vi "LVClasse_SurfaceFloatWithPupil Read SurfaceFloatWithPupil.vi"(8 "error in (no error)":errorcluster, 11 "SurfaceFloatWithPupil in":refnum<class "SurfaceFloatWithPupil.lvclass">) -> (0 "error out":errorcluster, 2 "SurfaceFloatWithPupil":T1, 3 "SurfaceFloatWithPupil out":refnum<class "SurfaceFloatWithPupil.lvclass">)   [LabVIEW 2020, in "SurfaceFloatWithPupil.lvclass"]
uses:
  SurfaceFloatWithPupil.lvclass
  ClassID.ctl
  SurfaceFloatWithPupil.lvclass/SurfaceFloatWithPupil.ctl
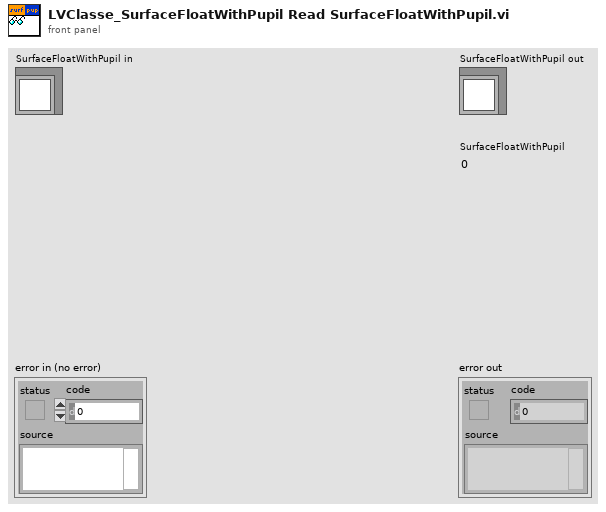
[diagram p1: front panel]
types:
  T1 = typedef "ClassID.ctl" = i64
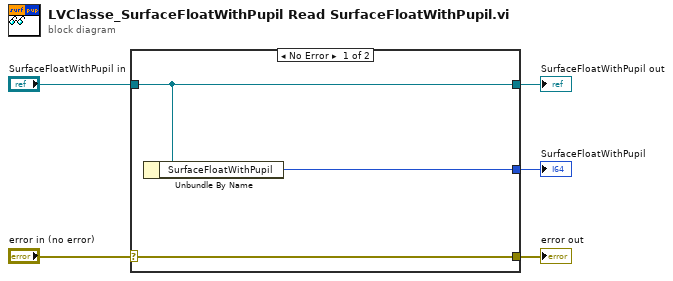
[diagram p0: block diagram]
diagram:
  n1 = case shown="No Error" "error in (no error)" {
    selector: "error in (no error)" -> [w8 w9]
    tunnel: [w8 w9] -> w4
    tunnel: [w7 w10] -> w2
    tunnel: "SurfaceFloatWithPupil in" -> [w7 w10]
    tunnel: [w6 _] -> w1
    frame No Error {
      n2 = Unbundle By Name(w7) -> ("SurfaceFloatWithPupil"=w6:T1)
    }
    frame Error {
    }
  }
  "error out" <- w4
  "SurfaceFloatWithPupil out" <- w2
  "SurfaceFloatWithPupil" <- w1
